vi "Configure Network Interface.vi"(8 "error in (no error)":errorcluster, 9 "network interface configuration":T1, 10 "hardware interface index":u16, 11 "PLBB in":refnum<class "PL BlackBox Modbus Client.lvclass">) -> (0 "error out":errorcluster, 3 "PLBB out":refnum<class "PL BlackBox Modbus Client.lvclass">)   [LabVIEW 2015, in "PL BlackBox Modbus Client.lvclass"]
doc: "Configures the network interface."
uses:
  PL BlackBox Modbus Client.lvclass
  <vilib>/plasmapper/PL Modbus Client/PL Modbus Client.lvclass
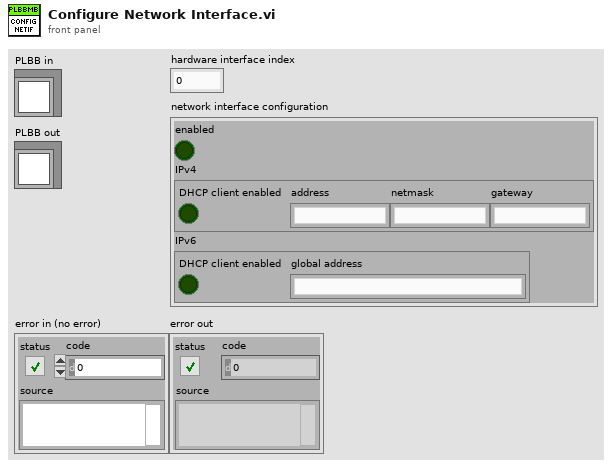
[diagram p1: front panel]
types:
  T1 = cluster{"enabled":bool, "IPv4":cluster{"DHCP client enabled":bool, "address":string, "netmask":string, "gateway":string}, "IPv6":cluster{"DHCP client enabled":bool, "global address":string}}
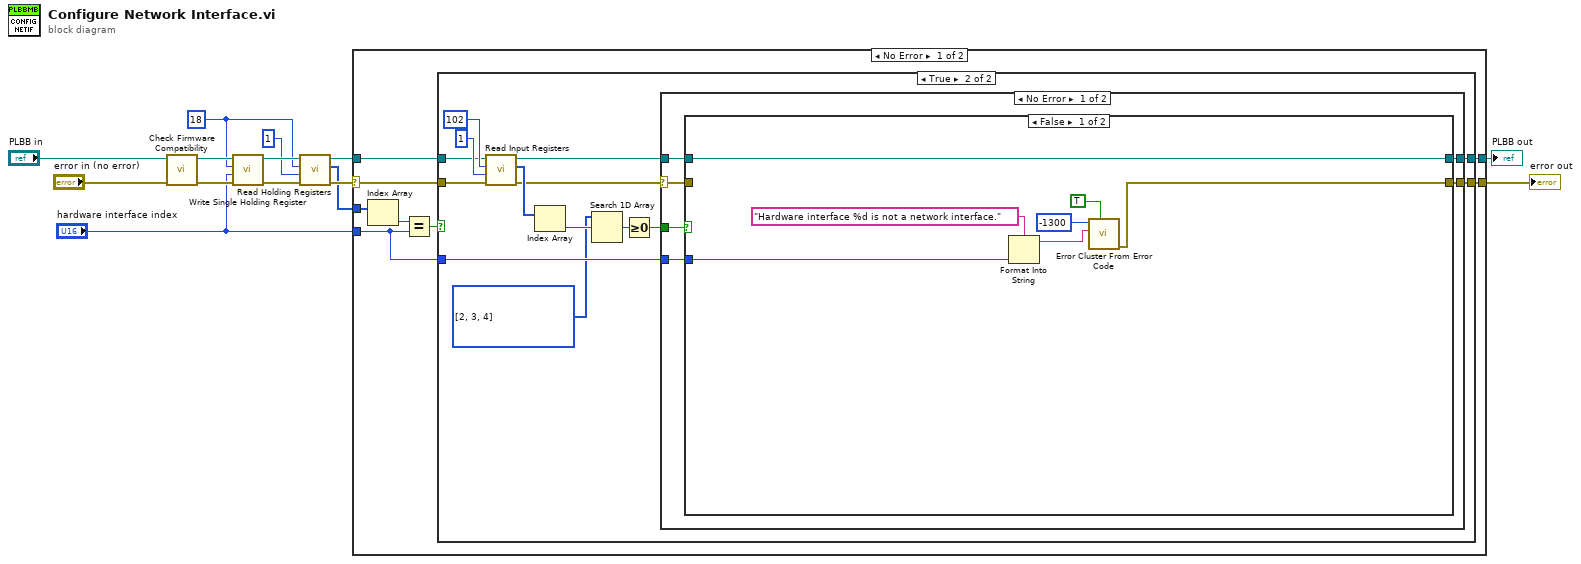
[diagram p0: block diagram]
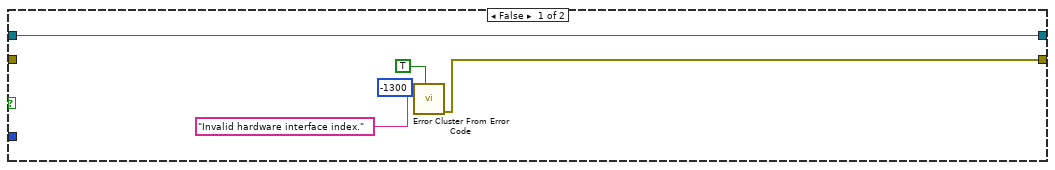
[diagram p2: hidden frame]
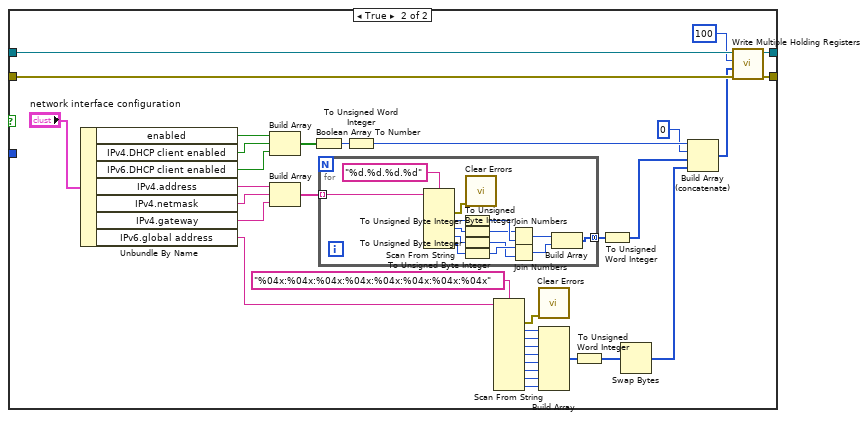
[diagram p3: hidden frame]
diagram:
  w6 = u16 18 ("address")
  n1 = call-dynamic "Check Firmware Compatibility.vi"("error in (no error)"="error in (no error)", "PLBB in"="PLBB in") -> ("error out"=w9:errorcluster, "PLBB out"=w10:refnum<class "PL BlackBox Modbus Client.lvclass">)  [unwired: 8 in]
  n2 = call <vilib>:"Write Single Holding Register.vi"("error in (no error)"=w9, "value"="hardware interface index", "address"=w6, "MODBUS in"=w10) -> ("error out"=w5:errorcluster, "MODBUS out"=w8:refnum<class "PL BlackBox Modbus Client.lvclass">)  [unwired: 6 in]
  n3 = call <vilib>:"Read Holding Registers.vi"("error in (no error)"=w5, "number of holding registers"=u16 1 ("address"), "address"=w6, "MODBUS in"=w8) -> ("error out"=w4:errorcluster, "values"=w2:u16[], "MODBUS out"=w3:refnum<class "PL BlackBox Modbus Client.lvclass">)  [unwired: 5 in]
  n4 = case shown="No Error" w4 {
    selector: w4 -> [w16 w105]
    tunnel: [w22 w105] -> w14
    tunnel: [w21 w106] -> w13
    tunnel: w3 -> [w17 w106]
    tunnel: w2 -> [w20 _]
    tunnel: "hardware interface index" -> [w15 _]
    frame No Error {
      n5 = Index Array(array=w20) -> (element=w19:u16)  [unwired: 1 in]
      n6 = Equal?(x=w19, y=w15) -> (x = y?=w18:bool)
      n7 = case shown="True" w18 {
        tunnel: [w23 w33] -> w22
        tunnel: [w27 w34] -> w21
        tunnel: w17 -> [w27 w39]
        tunnel: w16 -> [_ w38]
        tunnel: w15 -> [_ w32]
        frame False {
          n8 = call <vilib>:"Error Cluster From Error Code.vi"("show call chain? (False)"=TRUE, "error message (\"\")"="Invalid hardware interface index." ("error message (\"\")"), "error code (0)"=-1300) -> ("error out"=w23:errorcluster)  [unwired: 6 in]
        }
        frame True {
          w30 = u16[] [2, 3, 4] items=["Unknown", "UART", "Network interface", "Ethernet", "Wi-Fi"]
          n9 = call <vilib>:"Read Input Registers.vi"("error in (no error)"=w38, "number of input registers"=u16 1 ("address"), "address"=u16 102, "MODBUS in"=w39) -> ("error out"=w36:errorcluster, "values"=w37:u16[], "MODBUS out"=w35:refnum<class "PL BlackBox Modbus Client.lvclass">)  [unwired: 5 in]
          n10 = Index Array(array=w37) -> (element=w31:u16)  [unwired: 1 in]
          n11 = Search 1D Array(1D array=w30, element=w31) -> (index of element=w29:i32)  [unwired: 1 in]
          n12 = Greater Or Equal To 0?(x=w29) -> (x >= 0?=w28:bool)
          n13 = case shown="No Error" w36 {
            selector: w36 -> [w45 w103]
            tunnel: w28 -> [w47 _]
            tunnel: [w42 w104] -> w34
            tunnel: w35 -> [w46 w104]
            tunnel: [w43 w103] -> w33
            tunnel: w32 -> [w44 _]
            frame No Error {
              n14 = case shown="False" w47 {
                tunnel: w46 -> [w48 w85]
                tunnel: w45 -> [_ w86]
                tunnel: w44 -> [w51 _]
                tunnel: [w49 w87] -> w43
                tunnel: [w48 w88] -> w42
                frame False {
                  n15 = Format Into String(format string="Hardware interface %d is not a network interface." ("error message (\"\")"), w51) -> (resulting string=w50:string)  [unwired: 2 in, 1 out]
                  n16 = call <vilib>:"Error Cluster From Error Code.vi"("show call chain? (False)"=TRUE, "error message (\"\")"=w50, "error code (0)"=-1300) -> ("error out"=w49:errorcluster)  [unwired: 6 in]
                }
                frame True {
                  n17 = Unbundle By Name("network interface configuration") -> ("enabled"=w82:bool, "IPv4.DHCP client enabled"=w80:bool, "IPv6.DHCP client enabled"=w81:bool, "IPv4.address"=w77:string, "IPv4.netmask"=w75:string, "IPv4.gateway"=w76:string, "IPv6.global address"=w71:string)
                  n18 = Build Array(w82, w80, w81) -> (w79:bool[])
                  n19 = Build Array(w77, w75, w76) -> (w74:string[])
                  n20 = Boolean Array To Number(Boolean array=w79) -> (number=w78:u32)
                  n21 = for {
                    tunnel: w74 -> [w102] mode=indexing
                    tunnel: [w100] -> w73 mode=concatenating
                    n22 = Scan From String(format string="%d.%d.%d.%d", input string=w102) -> (error out=w97:errorcluster, output 1=w96:i32, output 2=w95:i32, output 3=w94:i32, output 4=w93:i32)  [unwired: 6 in, 2 out]
                    n23 = To Unsigned Byte Integer(number=w96) -> (unsigned 8bit integer=w92:u8)
                    n24 = To Unsigned Byte Integer(number=w95) -> (unsigned 8bit integer=w91:u8)
                    n25 = To Unsigned Byte Integer(number=w94) -> (unsigned 8bit integer=w89:u8)
                    n26 = To Unsigned Byte Integer(number=w93) -> (unsigned 8bit integer=w90:u8)
                    n27 = call <vilib>:"Clear Errors.vi"("error in (no error)"=w97) -> ()  [unwired: 5 in, 2 out]
                    n28 = Join Numbers(hi=w91, lo=w92) -> ((hi.lo)=w99:u16)
                    n29 = Join Numbers(hi=w90, lo=w89) -> ((hi.lo)=w98:u16)
                    n30 = Build Array(w99, w98) -> (w100:u16[])
                  }
                  n31 = To Unsigned Word Integer(number=w78) -> (unsigned 16bit integer=w56:u16)
                  n32 = Scan From String(format string="%04x:%04x:%04x:%04x:%04x:%04x:%04x:%04x", input string=w71) -> (error out=w61:errorcluster, output 1=w69:u32, output 2=w68:u32, output 3=w67:u32, output 4=w66:u32, output 5=w62:u32, output 6=w63:u32, output 7=w64:u32, output 8=w65:u32)  [unwired: 10 in, 2 out]
                  n33 = call <vilib>:"Clear Errors.vi"("error in (no error)"=w61) -> ()  [unwired: 5 in, 2 out]
                  n34 = Build Array(w69, w68, w67, w66, w62, w63, w64, w65) -> (w60:u32[])
                  n35 = To Unsigned Word Integer(number=w60) -> (unsigned 16bit integer=w58:u16[])
                  n36 = To Unsigned Word Integer(number=w73) -> (unsigned 16bit integer=w70:u16[])
                  n37 = Swap Bytes(anything=w58) -> (byte swapped=w57:u16[])
                  n38 = Build Array (concatenate)(w56, u16 0 ("element"), w70, w57) -> (w59:u16[])
                  n39 = call <vilib>:"Write Multiple Holding Registers.vi"("error in (no error)"=w86, "values"=w59, "address"=u16 100, "MODBUS in"=w85) -> ("error out"=w87:errorcluster, "MODBUS out"=w88:refnum<class "PL BlackBox Modbus Client.lvclass">)  [unwired: 6 in]
                }
              }
            }
            frame Error {
            }
          }
        }
      }
    }
    frame Error {
    }
  }
  "error out" <- w14
  "PLBB out" <- w13
